vi "Disconnect.vi"(8 "Error In":errorcluster, 11 "Nest Config":T1) -> (0 "Error Out":errorcluster)   [LabVIEW 2013, in "LVH-Nest.lvlib"]
doc: "Close the connection to the Nest server."
uses:
  LVH-Nest.lvlib
  Private/Type Defs/Nest Config.ctl
  <vilib>/httpClient/ClientHandle.ctl
  Private/Type Defs/Session Data.ctl
  <vilib>/httpClient/LabVIEWHTTPClient.lvlib
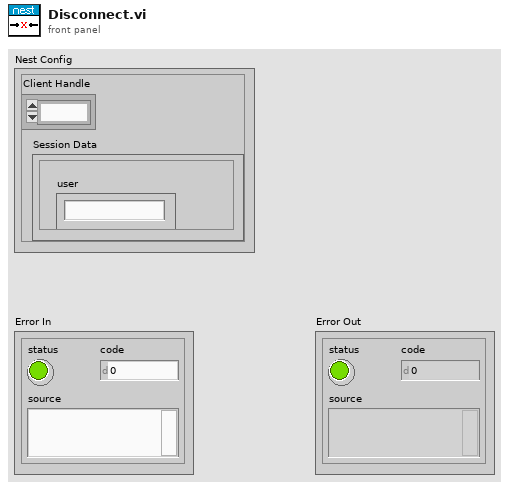
[diagram p1: front panel]
types:
  T1 = typedef "LVH-Nest.lvlib/Nest Config.ctl" = cluster{"Client Handle":T2, "Session Data":T3}
  T2 = typedef "LabVIEWHTTPClient.lvlib/ClientHandle.ctl" = refnum<k1>
  T3 = typedef "LVH-Nest.lvlib/Session Data.ctl" = cluster{"is_superuser":bool, "is_staff":bool, "urls":cluster{"transport_url":string, "rubyapi_url":string, "weather_url":string, "log_upload_url":string, "support_url":string}, "limits":cluster{"thermostats_per_structure":u32, "structures":u32, "thermostats":u32, "smoke_detectors":u32, "smoke_detectors_per_structure":u32}, "access_token":string, "userid":string, "expires_in":string, "email":string, "user":string, "language":string}
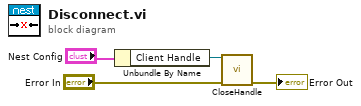
[diagram p0: block diagram]
diagram:
  n1 = Unbundle By Name("Nest Config") -> ("Client Handle"=w3:T2)
  n2 = call <vilib>:"CloseHandle.vi"("client handle"=w3, "error in (no error)"="Error In") -> ("error out"=→"Error Out":errorcluster)  [unwired: 13 in]
